vi "WriteAnalogLine.vi"(0 "Physical Channel(s)":tag="DAQ/ao0", 1 "Max Voltage":dbl=10.0, 2 "Min Voltage":dbl=-10.0, 3 "Voltage":dbl format="%0.2f") -> (6 "error out":errorcluster)   [LabVIEW 2012]
uses:
  <vilib>/DAQmx/write.llb/DAQmx Write (Analog DBL 1Chan 1Samp).vi
  <vilib>/DAQmx/create/channels.llb/DAQmx Create Channel (AO-Voltage-Basic).vi
  <vilib>/DAQmx/miscellaneous.llb/DAQmx Fill In Error Info.vi
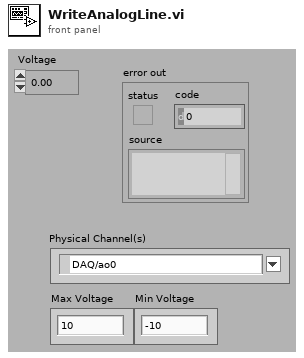
[diagram p1: front panel]
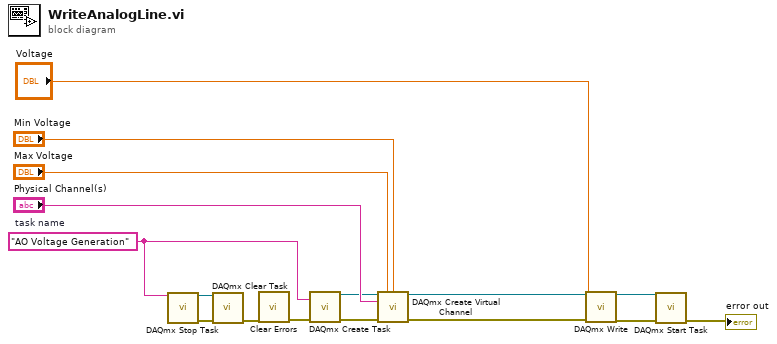
[diagram p0: block diagram]
diagram:
  w6 = "AO Voltage Generation"  # task name
  n1 = call <vilib>:"DAQmx Stop Task.vi"("task/channels in"=w6) -> ("task out"=w8:refnum<k21>, "error out"=w7:errorcluster)  [unwired: 13 in]
  n2 = call <vilib>:"DAQmx Clear Task.vi"("task in"=w8, "error in"=w7) -> ("error out"=w5:errorcluster)  [unwired: 13 in]
  n3 = call <vilib>:"Clear Errors.vi"("error in (no error)"=w5) -> ("error out"=w4:errorcluster)  [unwired: 6 in]
  n4 = call <vilib>:"DAQmx Create Task.vi"("new task name"=w6, "error in"=w4) -> ("task out"=w9:refnum<k21>, "error out"=w10:errorcluster)  [unwired: 12 in]
  n5 = call-poly <vilib>:"DAQmx Create Virtual Channel.vi"("task in"=w9, "maximum value"="Max Voltage", "minimum value"="Min Voltage", "physical channels"="Physical Channel(s)", "error in"=w10) -> ("task out"=w3:refnum<k21>, "error out"=w2:errorcluster)  [unwired: 9 in]
  n6 = call-poly <vilib>:"DAQmx Write.vi"("task/channels in"=w3, "data"="Voltage", "error in"=w2) -> ("task out"=w16:refnum<k21>, "error out"=w15:errorcluster)  [unwired: 10 in, 1 out]
  n7 = call <vilib>:"DAQmx Start Task.vi"("task/channels in"=w16, "error in"=w15) -> ("error out"=→"error out":errorcluster)  [unwired: 12 in, 1 out]
